vi "ScaleTo_dBm.vi"(11 "PowerIn (unscaled)":dbl[](array[numeric])) -> (3 "PowerOut (dBm)":dbl[](array[numeric]))   [LabVIEW 2018]
uses:
  Controls/Enums/ScaleMeasure.ctl
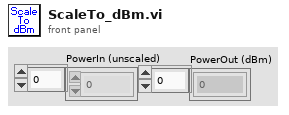
[diagram p1: front panel]
types:
  T1 = typedef "ScaleMeasure.ctl" = enum16{"1", "10", "50", "42"}
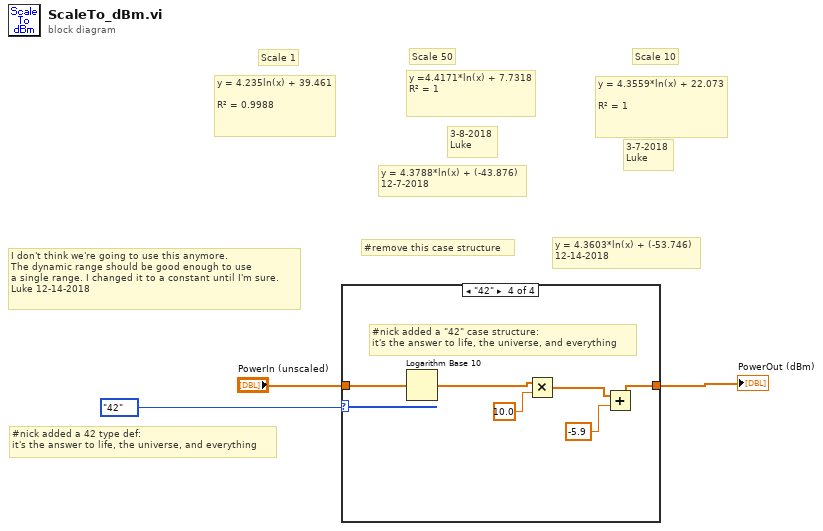
[diagram p0: block diagram]
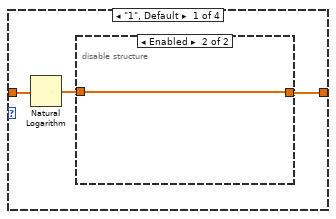
[diagram p2: hidden frame]
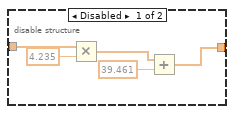
[diagram p3: hidden frame]
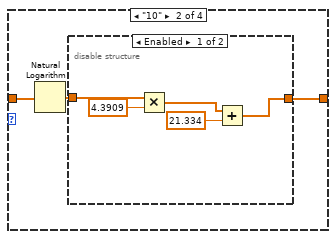
[diagram p4: hidden frame]
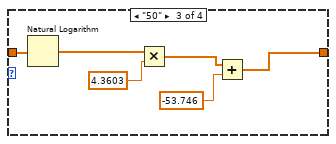
[diagram p6: hidden frame]
diagram:
  # "#nick added a 42 type def:\nit's the answer to life, the universe, and everything"
  # "y = 4.3603*ln(x) + (-53.746)\n12-14-2018"
  # "I don't think we're going to use this anymore.\nThe dynamic range should be good enough to use\na single range. I changed it to a constant until I'm sure.\nLuke 12-14-2018"
  # "y = 4.3788*ln(x) + (-43.876)\n12-7-2018"
  # "#remove this case structure"
  # "3-7-2018\nLuke"
  # "3-8-2018\nLuke"
  # "y = 4.235ln(x) + 39.461\n\nR² = 0.9988"
  # "y = 4.3559*ln(x) + 22.073\n\nR² = 1"
  # "Scale 10"
  # "Scale 1"
  # "Scale 50"
  # "y =4.4171*ln(x) + 7.7318\nR² = 1"
  n1 = case shown="\"42\"" ScaleMeasure."42" ("ScaleMeasEnum") {
    tunnel: "PowerIn (unscaled)" -> [w6 w15 w27 w33]
    tunnel: [w4 w14 w26 w28] -> w2
    frame "1", Default {
      n2 = Natural Logarithm(1:w6) -> (0:w5:dbl[])
      n3 = disable-structure shown="Enabled" {
        disable-tunnel: w5 -> [w11 w12]
        disable-tunnel: [w7 w12] -> w4
        frame Disabled {
          n4 = Multiply(x=w11, y=4.235) -> (x*y=w9:dbl[])
          n5 = Add(x=w9, y=39.461) -> (x+y=w7:dbl[])
        }
        frame Enabled {
        }
      }
    }
    frame "10" {
      n6 = Natural Logarithm(1:w15) -> (0:w13:dbl[])
      n7 = disable-structure shown="Enabled" {
        disable-tunnel: [w20 w21] -> w14
        disable-tunnel: w13 -> [w19 w21]
        frame Enabled {
          n8 = Multiply(x=w19, y=4.3909) -> (x*y=w17:dbl[])
          n9 = Add(x=w17, y=21.334) -> (x+y=w20:dbl[])
        }
        frame Disabled {
        }
      }
    }
    frame "50" {
      n10 = Natural Logarithm(1:w27) -> (0:w25:dbl[])
      n11 = Multiply(x=w25, y=4.3603) -> (x*y=w24:dbl[])
      n12 = Add(x=w24, y=-53.746) -> (x+y=w26:dbl[])
    }
    frame "42" {
      # "#nick added a \"42\" case structure:\nit's the answer to life, the universe, and everything"
      n13 = Logarithm Base 10(1:w33) -> (0:w29:dbl[])
      n14 = Multiply(x=w29, y=10.0) -> (x*y=w32:dbl[])
      n15 = Add(x=w32, y=-5.9) -> (x+y=w28:dbl[])
    }
  }
  "PowerOut (dBm)" <- w2
